vi "Send Contestant Buzzed.vi"(7 "Message Priority (Normal)":T1=enum."Normal", 8 "error in (no error)":errorcluster, 10 "Contestant":i32, 11 "Message Enqueuer":refnum<class "Message Enqueuer.lvclass">) -> (0 "error out":errorcluster, 3 "Message Enqueuer out":refnum<class "Message Enqueuer.lvclass">)   [LabVIEW 2024, in "MC Prompt.lvlib" / "Contestant Buzzed Msg.lvclass"]
doc: "This VI sends the message to an actor."
uses:
  Contestant Buzzed Msg.lvclass
  <vilib>/ActorFramework/Message Enqueuer/Message Enqueuer.lvclass
  <vilib>/ActorFramework/Message Enqueuer/Message Priority.ctl
  Applications/National Instruments/LabVIEW 2024 64-bit/vi.lib/ActorFramework/Message/Message.lvclass
  Contestant Buzzed Msg.lvclass/Contestant Buzzed Msg.ctl
  <vilib>/ActorFramework/Message Enqueuer/Message Enqueuer.lvclass/Message Enqueuer.ctl
  <vilib>/ActorFramework/Message Priority Queue/Priority Enqueue.vi
  Users/elijahkerry/challenge-of-champions/MC Prompt/MC Prompt Messages/Contestant Buzzed Msg/Contestant Buzzed Msg.lvclass
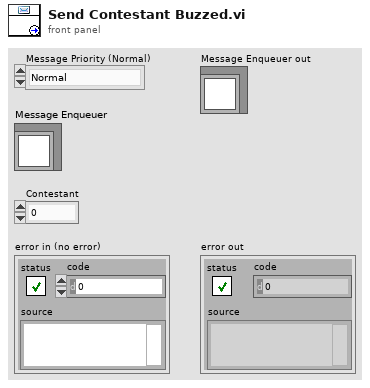
[diagram p1: front panel]
types:
  T1 = typedef "Actor Framework.lvlib/Message Enqueuer.lvclass/Message Priority.ctl" = enum16{"Low", "Normal", "High"}
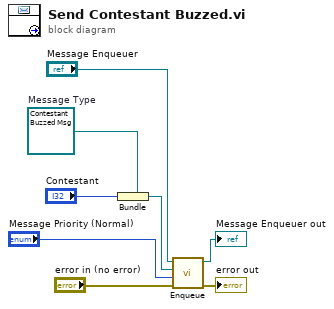
[diagram p0: block diagram]
diagram:
  w5 = refnum<class "Contestant Buzzed Msg.lvclass"> refnum  # Message Type
  n1 = Bundle(cluster=w5, "Contestant") -> (w4:refnum<class "Contestant Buzzed Msg.lvclass">)
  n2 = call <vilib>:"Enqueue.vi"("error in (no error)"="error in (no error)", "Message Priority (Normal)"="Message Priority (Normal)", "Message"=w4, "Message Enqueuer in"="Message Enqueuer") -> ("error out"=→"error out":errorcluster, "Message Enqueuer in"=→"Message Enqueuer out":refnum<class "Message Enqueuer.lvclass">)  [unwired: 6 in]
